vi "Get Rx Hardware Channel Data.vi"(8 "error in":errorcluster, 11 "custom device ref in":T1 format="%.0x") -> (0 "error out":errorcluster, 1 "Rx hardware channel data":T2[](array[typedef]) {"labels settings for RT"."Label Timestamp Channel Data Reference" format="%.0x"; "labels settings for RT"."Word Initial Raw Value" format="%032.0f"; "labels settings for RT"."Label Disable/Trigger Channel Reference" format="%.0x"; "labels settings for RT"."parameter driver data"."Tx parameter refs" format="%.0x"; "labels settings for RT"."SDI" format="%02b"; "labels settings for RT"."label" format="%.0o"}, 2 "incoming channels":T1[](array[typedef]) format="%.0x", 3 "custom device ref out":T1 format="%.0x", 5 "timing channel offset":i64)   [LabVIEW 2020]
uses:
  <vilib>/NI VeriStand/Custom Device API/Custom Device Item Ref.ctl
  RT Hardware Channel Settings.ctl
  RT Label Settings.ctl
  Label.ctl
  RT Parameters.ctl
  Parameter Definition.ctl
  <vilib>/NI/NI VeriStand Encoding and Decoding/Encoding.ctl
  Transfer Type.ctl
  <vilib>/NI VeriStand/Custom Device API/Data Reference.ctl
  Transfer Speed.ctl
  <vilib>/NI VeriStand/Custom Device API/Custom Device API.lvlib
  <vilib>/NI/NI VeriStand Encoding and Decoding/Encoding and Decoding.lvlib
  Scripting/AIM/AIM ARINC 429 Scripting.lvlib
  Engine/Implementation/Execution Unit Factory/Execution Unit Factory.lvclass
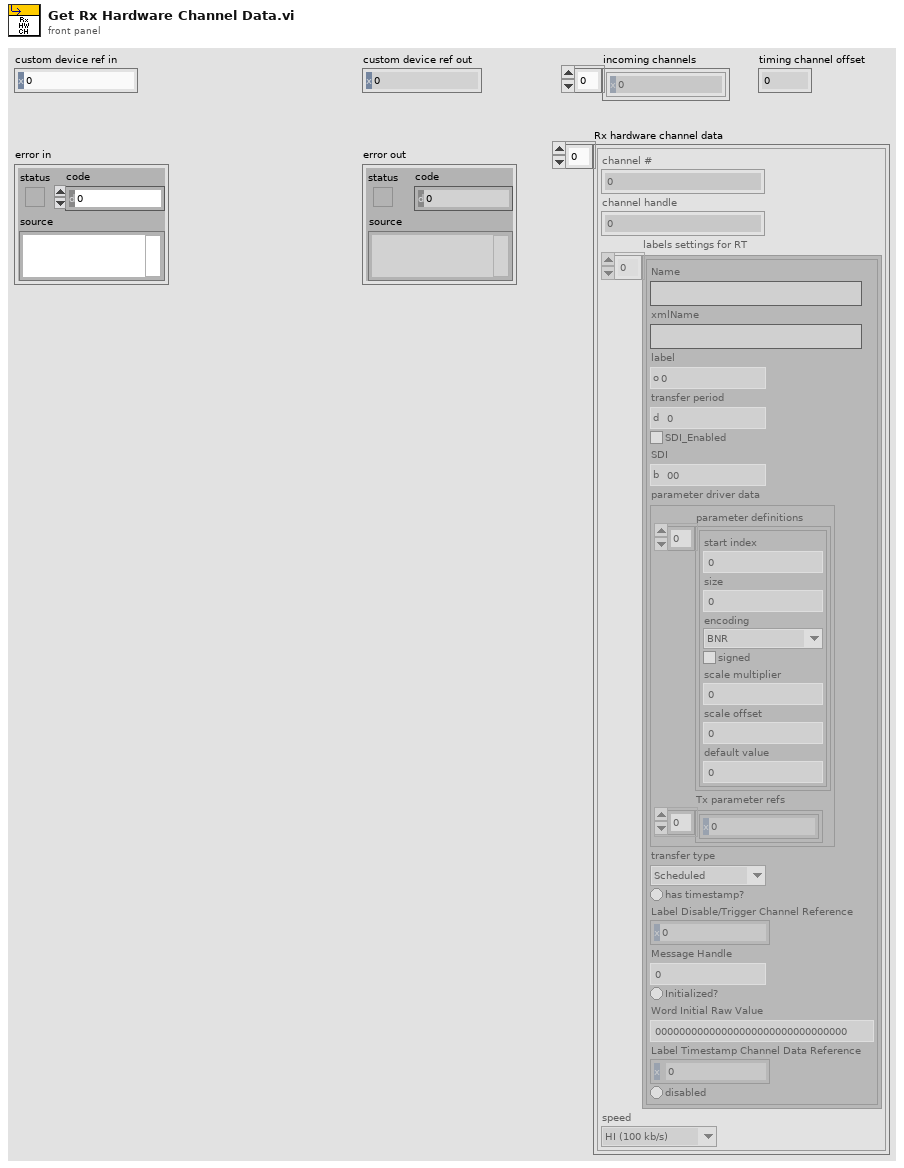
[diagram p1: front panel]
types:
  T1 = typedef "Custom Device API.lvlib/Custom Device Item Ref.ctl" = u64
  T2 = typedef "RT Hardware Channel Settings.ctl" = cluster{"channel #":u16, "channel handle":u64, "labels settings for RT":T3[], "speed":T10}
  T3 = typedef "RT Label Settings.ctl" = cluster{"Name":string, "xmlName":string, "label":T4, "transfer period":u32, "SDI_Enabled":bool, "SDI":u8, "parameter driver data":T5, "transfer type":T8, "has timestamp?":bool, "Label Disable/Trigger Channel Reference":T1, "Message Handle":u64, "Initialized?":bool, "Word Initial Raw Value":u32, "Label Timestamp Channel Data Reference":T9, "disabled":bool}
  T4 = typedef "Label.ctl" = u8
  T5 = typedef "RT Parameters.ctl" = cluster{"parameter definitions":T6[], "Tx parameter refs":T1[]}
  T6 = typedef "Parameter Definition.ctl" = cluster{"start index":i32, "size":i32, "encoding":T7, "signed":bool, "scale multiplier":dbl, "scale offset":dbl, "default value":dbl}
  T7 = typedef "Encoding and Decoding.lvlib/Encoding.ctl" = enum16{"BNR", "BCD", "Discrete"}
  T8 = typedef "Transfer Type.ctl" = enum16{"Scheduled", "Acyclic", "Block", "Strobe"}
  T9 = typedef "Custom Device API.lvlib/Data Reference.ctl" = i32
  T10 = typedef "Transfer Speed.ctl" = enum16{"LO (12.5 kb/s)", "HI (100 kb/s)"}
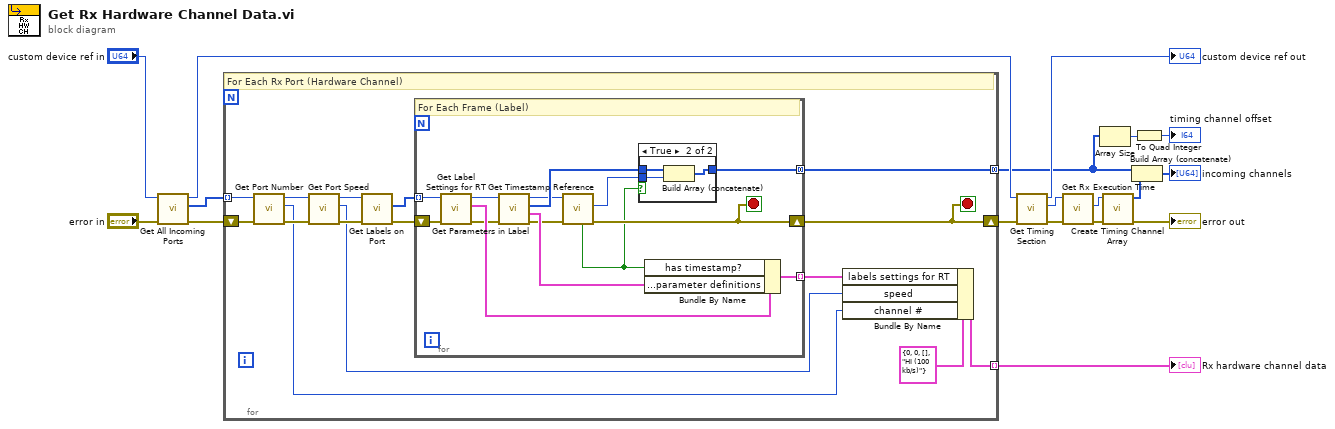
[diagram p0: block diagram]
diagram:
  n1 = call "Get All Incoming Ports.vi"("error in"="error in", "custom device ref"="custom device ref in") -> ("error out"=w15:errorcluster, "incoming ports"=w14:T1[], "custom device ref out"=w11:T1)  [unwired: 7 in]
  n2 = for {
    shift-right: [w32] -> w12
    shift-left: w15 -> [w27]
    tunnel: w14 -> [w28] mode=indexing
    tunnel: [w31] -> w16 mode=indexing
    tunnel: [w24] -> w5 mode=concatenating
    stop <- w32 stop-if-true
    # "For Each Rx Port (Hardware Channel)"
    n3 = call "Get Port Number.vi"("error in"=w27, "port ref"=w28) -> ("error out"=w23:errorcluster, "port number"=w19:u16, "port ref out"=w22:T1)  [unwired: 6 in, 1 out]
    n4 = call "Get Port Speed.vi"("error in"=w23, "port ref"=w22) -> ("error out"=w21:errorcluster, "speed"=w18:T10, "port ref out"=w20:T1)  [unwired: 7 in]
    n5 = call "Get Labels on Port.vi"("error in"=w21, "port ref"=w20) -> ("error out"=w25:errorcluster, "labels"=w26:T1[])  [unwired: 6 in, 2 out]
    n6 = for {
      tunnel: w26 -> [w46] mode=indexing
      shift-right: [w34] -> w32
      shift-left: w25 -> [w45]
      tunnel: [w42] -> w30 mode=indexing
      tunnel: [w39] -> w24 mode=concatenating
      stop <- w34 stop-if-true
      # "For Each Frame (Label)"
      n7 = call "Get Label Settings for RT.vi"("error in"=w45, "label ref in"=w46) -> ("error out"=w37:errorcluster, "label settings for RT"=w44:T3, "label ref out"=w38:T1)  [unwired: 7 in]
      n8 = call "Get Parameters in Label.vi"("error in"=w37, "label ref"=w38) -> ("error out"=w35:errorcluster, "parameter definitions"=w43:T6[], "parameters"=w41:T1[], "label ref out"=w36:T1)  [unwired: 6 in]
      n9 = call "Get Timestamp Reference.vi"("error in"=w35, "label ref"=w36) -> ("error out"=w34:errorcluster, "timestamp channel reference"=w40:T1, "timestamp channel found?"=w33:bool)  [unwired: 6 in, 1 out]
      n10 = case shown="True" w33 {
        tunnel: w41 -> [w47 w50]
        tunnel: w40 -> [_ w49]
        tunnel: [w47 w48] -> w39
        frame False {
        }
        frame True {
          n11 = Build Array (concatenate)(w50, w49) -> (w48:T1[])
        }
      }
      n12 = Bundle By Name(cluster=w44, "has timestamp?"=w33, "parameter driver data.parameter definitions"=w43) -> (w42:T3)
    }
    n13 = Bundle By Name(cluster=T2 {"channel #"=0, "channel handle"=0, "labels settings for RT"=[], "speed"=enum."HI (100 kb/s)"} ("RT hardware channel"), "labels settings for RT"=w30, "speed"=w18, "channel #"=w19) -> (w31:T2)
  }
  "Rx hardware channel data" <- w16
  n14 = call "Get Timing Section.vi"("error in"=w12, "custom device ref"=w11) -> ("error out"=w9:errorcluster, "timing"=w8:T1, "custom device ref out"=→"custom device ref out":T1)  [unwired: 6 in, 1 out]
  n15 = call "Get Rx Execution Time.vi"("error in"=w9, "timing ref"=w8) -> ("error out"=→"error out":errorcluster, "rx execution time ref"=w2:T1)  [unwired: 7 in, 1 out]
  n16 = Array Size(array=w5) -> (size(s)=w4:i32)
  n17 = call "Create Timing Channel Array.vi"("timing channel ref"=w2) -> ("timing channel ref array"=w1:T1[])  [unwired: 9 in, 1 out]
  n18 = Build Array (concatenate)(w5, w1) -> (→"incoming channels":T1[])
  n19 = To Quad Integer(1:w4) -> (0:→"timing channel offset":i64)
